vi "LWXPS_PositionerCompensationSpatialPeriodicNotchsSet.vi"(0 "Spatial Notch Bandwidth 1":dbl, 1 "Spatial Notch Gain 1":dbl, 2 "Spatial Notch Step 2":dbl, 3 "Spatial Notch Bandwidth 2":dbl, 4 "Spatial Notch Gain 2":dbl, 5 "Spatial Notch Step 3":dbl, 6 "Spatial Notch Step 1":dbl, 7 "Spatial Notch Bandwidth 3":dbl, 8 "Positioner Name":string, 9 "Spatial Notch Gain 3":dbl, 10 "XPS Reference IN":refnum<k24>, 11 "LabVIEW error IN":errorcluster) -> (14 "XPS Reference OUT":refnum<k24>, 15 "Returned error code":i32, 18 "XPS Error String":string, 19 "LabVIEW error OUT":errorcluster)   [LabVIEW 2014]
uses:
  D:/XPSQ8_LabView_Library/Development/Source/Dll/Newport.XPS.CommandInterface.dll
  Dll/Newport.XPS.CommandInterface.dll
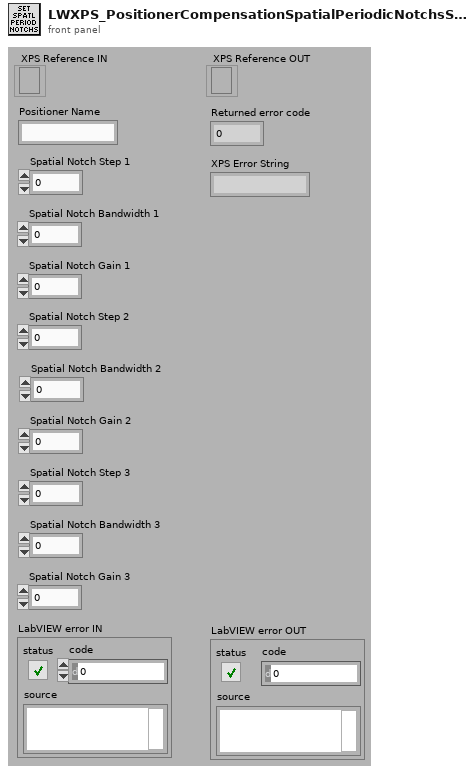
[diagram p1: front panel]
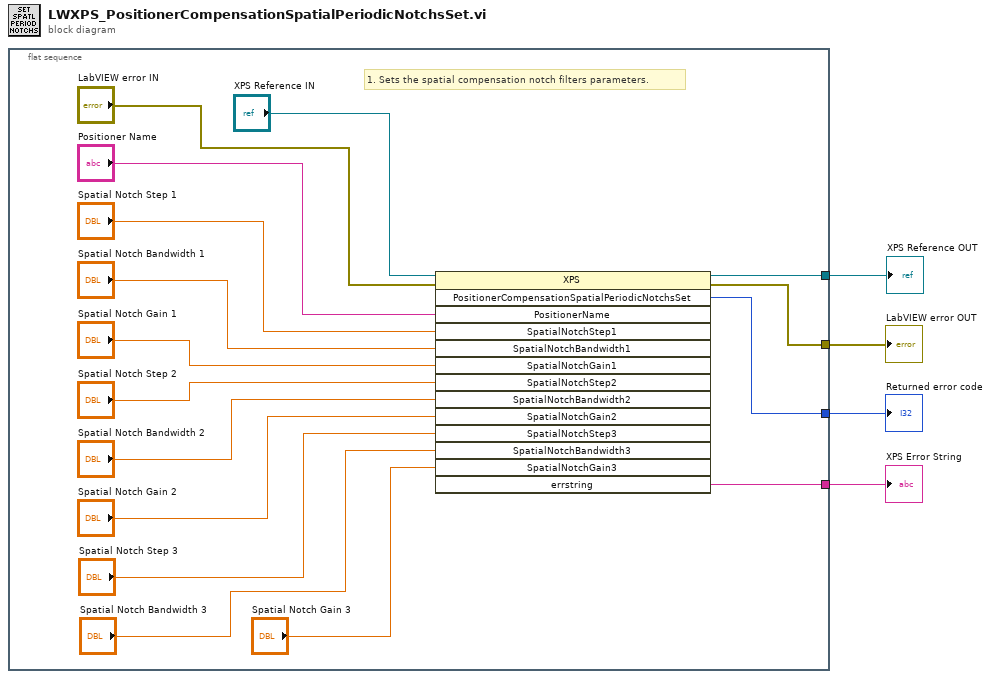
[diagram p0: block diagram]
diagram:
  n1 = flat-sequence {
    tunnel: [w16] -> w4
    tunnel: [w19] -> w3
    tunnel: [w18] -> w2
    tunnel: [w7] -> w1
    frame #0 {
      # "1. Sets the spatial compensation notch filters parameters."
      n2 = invoke class="XPS" method="PositionerCompensationSpatialPeriodicNotchsSet"(reference="XPS Reference IN", error in="LabVIEW error IN", "PositionerName"="Positioner Name", "SpatialNotchStep1"="Spatial Notch Step 1", "SpatialNotchBandwidth1"="Spatial Notch Bandwidth 1", "SpatialNotchGain1"="Spatial Notch Gain 1", "SpatialNotchStep2"="Spatial Notch Step 2", "SpatialNotchBandwidth2"="Spatial Notch Bandwidth 2", "SpatialNotchGain2"="Spatial Notch Gain 2", "SpatialNotchStep3"="Spatial Notch Step 3", "SpatialNotchBandwidth3"="Spatial Notch Bandwidth 3", "SpatialNotchGain3"="Spatial Notch Gain 3") -> (reference out=w16:refnum<k24>, error out=w19:errorcluster, "PositionerCompensationSpatialPeriodicNotchsSet"=w18:i32, "errstring"=w7:string)  [unwired: 2 in, 10 out]
    }
  }
  "XPS Error String" <- w1
  "XPS Reference OUT" <- w4
  "LabVIEW error OUT" <- w3
  "Returned error code" <- w2
